vi "下载程序.vi"(11 "boot?":bool) -> ()   [LabVIEW 2018]
uses:
  user32.dll
panel:
  out "布尔":bool
  # "程序下载中……"
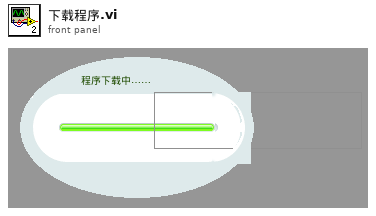
[diagram p1: front panel]
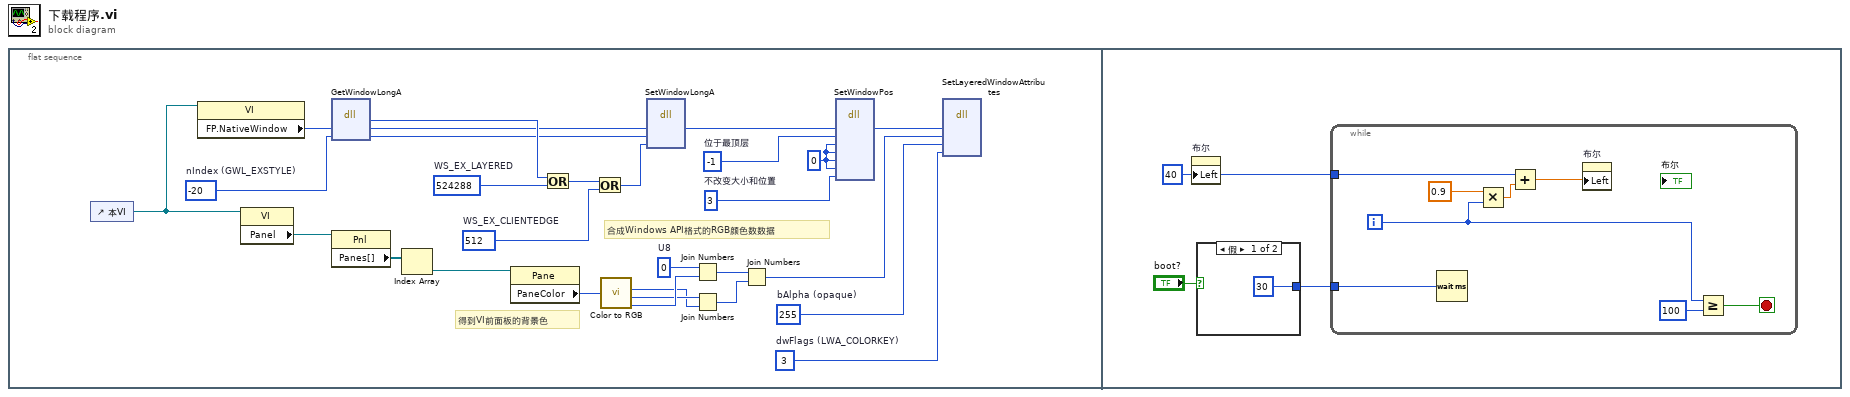
[diagram p0: block diagram]
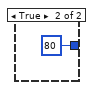
[diagram p2: hidden frame]
diagram:
  n1 = flat-sequence {
    frame #0 {
      w25 = 512  # WS_EX_CLIENTEDGE
      w21 = 3  # 不改变大小和位置
      w24 = 0 ("nIndex")
      w20 = -1  # 位于最顶层
      w2 = 255  # bAlpha (opaque)
      w1 = 3  # dwFlags (LWA_COLORKEY)
      w9 = u8 0  # U8
      w17 = 524288  # WS_EX_LAYERED
      w18 = -20  # nIndex (GWL_EXSTYLE)
      # "合成Windows API格式的RGB颜色数数据"
      # "得到VI前面板的背景色"
      n2 = control-ref of="本VI"() -> (w28:refnum<vi>)
      n3 = property class="VI"(reference=w28) -> ("FP.NativeWindow"=w19:u64)  [unwired: 1 in, 2 out]
      n4 = property class="VI"(reference=w28) -> ("Panel"=w4:refnum<vi>)  [unwired: 1 in, 2 out]
      n5 = dll-call lib="user32.dll" fn="GetWindowLongA"("handle"=w19, "nIndex"=w18) -> ("返回类型"=w16:i32, "handle"=w15:i32, "nIndex"=w14:i32)  [unwired: 3 in, 2 out]
      n6 = property class="Pnl"(reference=w4) -> ("Panes[]"=w5:refnum<vi>[])  [unwired: 1 in, 2 out]
      n7 = Index Array(array=w5) -> (element=w6:refnum<vi>)  [unwired: 1 in]
      n8 = property class="Pane"(reference=w6) -> ("PaneColor"=w10:u32)  [unwired: 1 in, 2 out]
      n9 = Or(x=w16, y=w17) -> (x .or. y?=w26:i32)
      n10 = Or(x=w26, y=w25) -> (x .or. y?=w27:i32)
      n11 = call <vilib>:"Color to RGB.vi"("Color"=w10) -> ("R"=w11:u8, "G"=w12:u8, "B"=w13:u8)  [unwired: 1 out]
      n12 = dll-call lib="USER32.DLL" fn="SetWindowLongA" label="SetWindowLong"("handle"=w15, "nIndex"=w14, "dwNewLong"=w27) -> ("handle"=w22:i32)  [unwired: 5 in, 3 out]
      n13 = Join Numbers(hi=w9, lo=w13) -> ((hi.lo)=w8:u16)
      n14 = Join Numbers(hi=w12, lo=w11) -> ((hi.lo)=w7:u16)
      n15 = Join Numbers(hi=w8, lo=w7) -> ((hi.lo)=w3:u32)
      n16 = dll-call lib="USER32.DLL" fn="SetWindowPos"("hWnd"=w22, "hWndInsertAfter"=w20, "x"=w24, "y"=w24, "cx"=w24, "cy"=w24, "wFlags"=w21) -> ("hWnd"=w23:i32)  [unwired: 9 in, 3 out]
      n17 = dll-call lib="USER32.DLL" fn="SetLayeredWindowAttributes" label="SetLayerdWindowAttributs"("handle"=w23, "crkey"=w3, "bAlpha"=w2, "dwFlags"=w1) -> ()  [unwired: 7 in, 3 out]
    }
    frame #1 {
      w31 = 40 ("位置:居左")
      n18 = property on="布尔" class="Bool (严格)"("Left"=w31) -> ()  [unwired: 2 in, 2 out]
      n19 = case shown="假" "boot?" {
        tunnel: [u32 30 ("等待时间（毫秒）") u32 80 ("等待时间（毫秒）")] -> w30
        frame False {
        }
        frame True {
        }
      }
      n20 = while {
        tunnel: w31 -> [w39]
        tunnel: w30 -> [w34]
        i -> [w37]
        stop <- w41 stop-if-true
        n21 = Wait (ms)(milliseconds to wait=w34) -> ()  [unwired: 1 out]
        n22 = Multiply(x=0.9, y=w37) -> (x*y=w38:dbl)
        n23 = Add(x=w39, y=w38) -> (x+y=w35:dbl)
        n24 = property on="布尔" class="Bool (严格)"("Left"=w35) -> ()  [unwired: 2 in, 2 out]
        n25 = Greater Or Equal?(x=w37, y=100) -> (x >= y?=w41:bool)
      }
    }
  }
